vi "PCO_ConvertSetFilter.vi"(8 "error in (no error)":errorcluster {"code" format="%x"}, 10 "strFilter":T1, 11 "ph":u64) -> (0 "error out":errorcluster {"code" format="%x"}, 2 "ErrorMessage":i32 format="%x", 3 "ph out":u64)   [LabVIEW 2020, in "Convert.lvlib"]
doc: "int PCOCONVERT_API PCO_ConvertSetFilter(HANDLE ph, PCO_Filter* pstrFilter);"
uses:
  Convert.lvlib
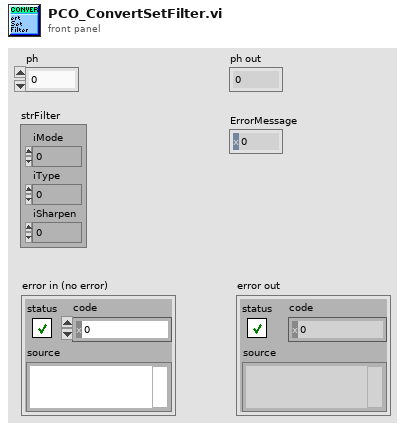
[diagram p1: front panel]
types:
  T1 = cluster{"iMode":i32, "iType":i32, "iSharpen":i32}
  T2 = cluster{"wSize":u16, "wDummy":u16, "iMode":i32, "iType":i32, "iSharpen":i32, "dwzzDummy1":cluster{u32, u32, u32, u32, u32, u32, u32, u32, u32, u32, u32, u32, u32, u32, u32, u32, u32, u32, u32, u32, u32, u32, u32, u32, u32, u32, u32, u32, u32, u32, u32, u32, u32, u32, u32, u32, u32, u32, u32, u32, u32, u32, u32, u32, u32, u32, u32, u32, u32, u32, u32, u32, u32, u32, u32, u32, u32, u32, u32, u32}}
  T3 = cluster{u32, u32, u32, u32, u32, u32, u32, u32, u32, u32, u32, u32, u32, u32, u32, u32, u32, u32, u32, u32, u32, u32, u32, u32, u32, u32, u32, u32, u32, u32, u32, u32, u32, u32, u32, u32, u32, u32, u32, u32, u32, u32, u32, u32, u32, u32, u32, u32, u32, u32, u32, u32, u32, u32, u32, u32, u32, u32, u32, u32}
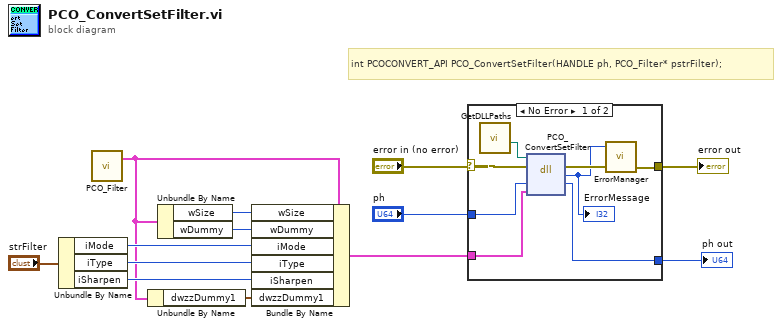
[diagram p0: block diagram]
diagram:
  # "int PCOCONVERT_API PCO_ConvertSetFilter(HANDLE ph, PCO_Filter* pstrFilter);"
  n1 = Unbundle By Name("strFilter") -> ("iMode"=w8:i32, "iType"=w7:i32, "iSharpen"=w6:i32)
  n2 = call "PCO_Filter.vi"() -> ("PCO_Filter_Raw"=w2:T2)  [unwired: 4 in, 3 out]
  n3 = Unbundle By Name(w2) -> ("dwzzDummy1"=w5:T3)
  n4 = Unbundle By Name(w2) -> ("wSize"=w4:u16, "wDummy"=w3:u16)
  n5 = Bundle By Name(cluster=w2, "wSize"=w4, "wDummy"=w3, "iMode"=w8, "iType"=w7, "iSharpen"=w6, "dwzzDummy1"=w5) -> (w1:T2)
  n6 = case shown="No Error" "error in (no error)" {
    selector: "error in (no error)" -> [w18 w23]
    tunnel: "ph" -> [w21 w22]
    tunnel: [w20 w22] -> w12
    tunnel: w1 -> [w19 _]
    tunnel: [w16 w23] -> w11
    frame No Error {
      n7 = call "GetDLLPaths.vi"() -> ("PCO_Conv_Path"=w14:path)  [unwired: 9 in, 2 out]
      n8 = dll-call lib="?" fn="PCO_ConvertSetFilter"(path in=w14, error in=w18, "ph"=w21, "pstrFilter"=w19) -> (error out=w17:errorcluster, "return type"=w15:i32, "ph"=w20:u64)  [unwired: 2 in, 1 out]
      "ErrorMessage" <- w15
      n9 = call "ErrorManager.vi"("error in (no error)"=w17, "error code"=w15) -> ("error out"=w16:errorcluster)  [unwired: 3 in]
    }
    frame Error {
    }
  }
  "ph out" <- w12
  "error out" <- w11
